vi "sabertooth packetized settings.vi"(1 "Value (Data)":u8, 2 "Setting (Command)":u8(ring)=15 items=["Min Voltage"=2, "Max Voltage"=3, "Serial Timeout"=14, "Baud Rate"=15, "Ramping"=16, "Deadband"=17], 3 "Sabertooth Addresses":T1=128 items=["Sabertooth 1"=128, "Sabertooth 2"=129, "Sabertooth 3"=130, "Sabertooth 4"=131, "Sabertooth 5"=132, "Sabertooth 6"=133, "Sabertooth 7"=134, "Sabertooth 8"=135]) -> (0 "Uart Write Message":string)   [LabVIEW 2018]
uses:
  package/Sabertooth Address Select.ctl
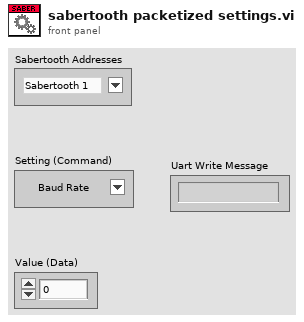
[diagram p1: front panel]
types:
  T1 = typedef "Sabertooth Address Select.ctl" = u8
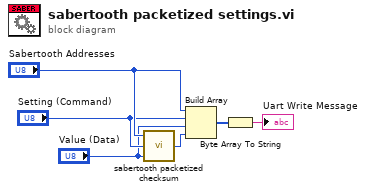
[diagram p0: block diagram]
diagram:
  n1 = call "sabertooth packetized checksum.vi"("Data"="Value (Data)", "Command"="Setting (Command)", "Address"="Sabertooth Addresses") -> ("Checksum"=w3:u8)
  n2 = Build Array("Sabertooth Addresses", "Setting (Command)", "Value (Data)", w3) -> (w2:T1[])
  n3 = Byte Array To String(unsigned byte array=w2) -> (string=→"Uart Write Message":string)
